vi "SMPS Calc IV.vi"(7 "Init?":bool, 10 "IV in":sgl[](array[numeric]), 11 "DMA in":refnum<class "DMA.lvclass">) -> (2 "IV out":sgl[](array[numeric]), 3 "DMA out":refnum<class "DMA.lvclass">)   [LabVIEW 2015, in "DMA.lvclass"]
uses:
  DMA.lvclass
  DMA.lvclass/DMA.ctl
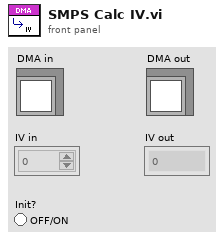
[diagram p1: front panel]
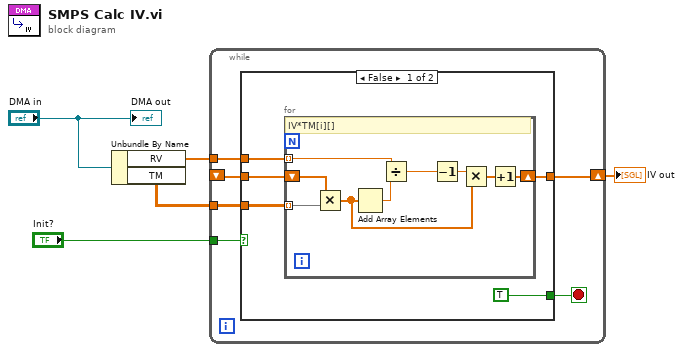
[diagram p0: block diagram]
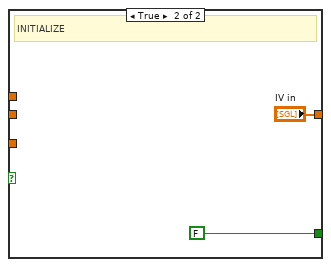
[diagram p2: hidden frame]
diagram:
  n1 = Unbundle By Name("DMA in") -> ("RV"=w4:sgl[], "TM"=w3:sgl[][])
  n2 = while {
    tunnel: w4 -> [w11]
    tunnel: w3 -> [w10]
    tunnel: "Init?" -> [w8]
    shift-right: [w9] -> w2
    shift-left: _ -> [w7]
    stop <- w6 stop-if-true
    n3 = case shown="False" w8 {
      tunnel: w11 -> [w16 _]
      tunnel: w10 -> [w15 _]
      tunnel: [w14 "IV in"] -> w9
      tunnel: w7 -> [w12 _]
      tunnel: [TRUE FALSE] -> w6
      frame False {
        n4 = for {
          tunnel: w15 -> [w24] mode=indexing
          tunnel: w16 -> [w23] mode=indexing
          shift-right: [w17] -> w14
          shift-left: w12 -> [w25]
          # "IV*TM[i][]"
          n5 = Multiply(x=w25, y=w24) -> (x*y=w19:sgl[])
          n6 = Add Array Elements(numeric array=w19) -> (sum=w22:sgl)
          n7 = Divide(x=w23, y=w22) -> (x/y=w21:sgl)
          n8 = Decrement(x=w21) -> (x-1=w20:sgl)
          n9 = Multiply(x=w20, y=w19) -> (x*y=w18:sgl[])
          n10 = Increment(x=w18) -> (x+1=w17:sgl[])
        }
      }
      frame True {
        # "INITIALIZE"
      }
    }
  }
  "IV out" <- w2
  "DMA out" <- "DMA in"
